vi "Read ADC.vi"(8 "error in (no error)":errorcluster, 10 "ADC canal":dbl, 11 "Cypress in":refnum<class "Cypress.lvclass">) -> (0 "error out":errorcluster, 3 "Cypress out":refnum<class "Cypress.lvclass">)   [LabVIEW 2020, in "Cypress.lvclass"]
doc: "Método heredado del padre con un override"
uses:
  Cypress.lvclass
  927a9c60-a38c-4387-bcea-af75955b7cfb.vi
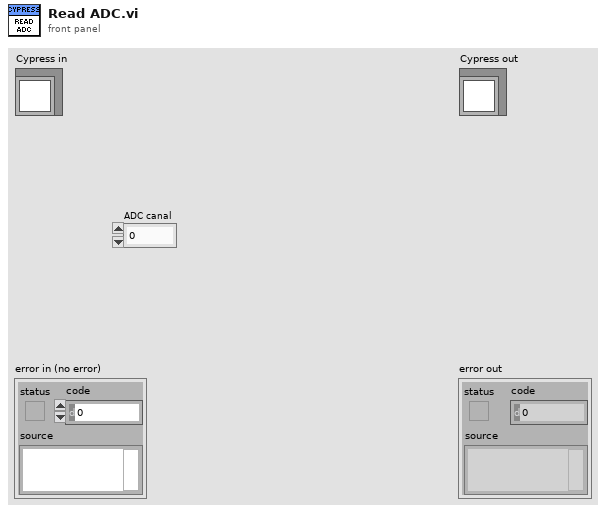
[diagram p1: front panel]
types:
  T1 = typedef "Serial device.lvclass/Brand combobox.ctl" = string
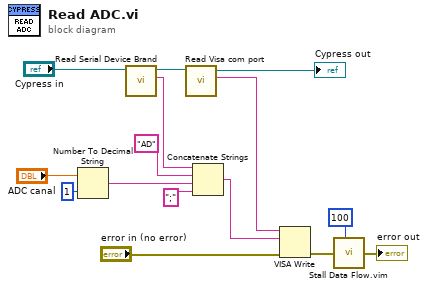
[diagram p0: block diagram]
diagram:
  n1 = Number To Decimal String(number="ADC canal", width (-)=i16 1) -> (decimal integer string=w9:string)
  n2 = call-dynamic "Read Serial Device Brand.vi"("Serial device in"="Cypress in") -> ("Serial Device Brand"=w11:T1, "Serial device out"=w15:refnum<class "Cypress.lvclass">)  [unwired: 8 in, 1 out]
  n3 = call-dynamic "Read Visa com port.vi"("Serial device in"=w15) -> ("Visa com port"=w7:string, "Serial device out"=→"Cypress out":refnum<class "Cypress.lvclass">)  [unwired: 8 in, 1 out]
  n4 = Concatenate Strings(w11, "AD" ("string"), w9, ";" ("string")) -> (w4:string)
  n5 = VISA Write(VISA resource name=w7, write buffer=w4, error in (no error)="error in (no error)") -> (error out=w5:errorcluster)  [unwired: 2 out]
  n6 = call "Stall Data Flow.vim"("value in"=w5, "milliseconds to wait"=u32 100) -> ("value out"=→"error out":errorcluster)  [unwired: 1 out]
